vi "robot - Draw Span.vi"(4 "Color":u32(colorbox)=10079334, 6 "Center 2":cluster{"X":dbl, "Y":dbl}={"X"=50.0, "Y"=20.0}, 7 "Enhance Style":bool=TRUE, 8 "Center 1":cluster{"X":dbl, "Y":dbl}={"X"=20.0, "Y"=20.0}, 9 "Light Direction":dbl(knob)=314.8880943229338 scale=0.0..360.0 scale format="%.1f", 10 "Circle Spec":cluster{"Angle":dbl, "Height":dbl, "Ratio":dbl}={"Angle"=0.0, "Height"=10.0, "Ratio"=1.0}, 11 "Picture In":picture) -> (3 "Picture Out":picture)   [LabVIEW 2023]
doc: "Draw a single arm segment for the robot arm."
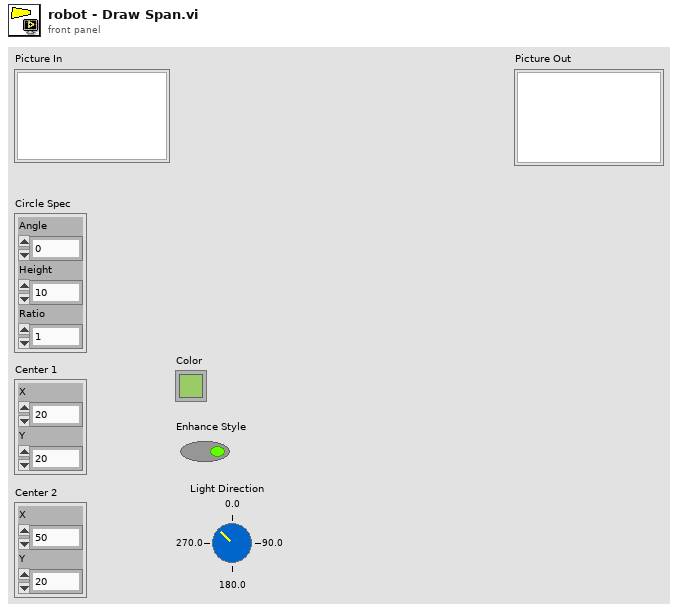
[diagram p1: front panel]
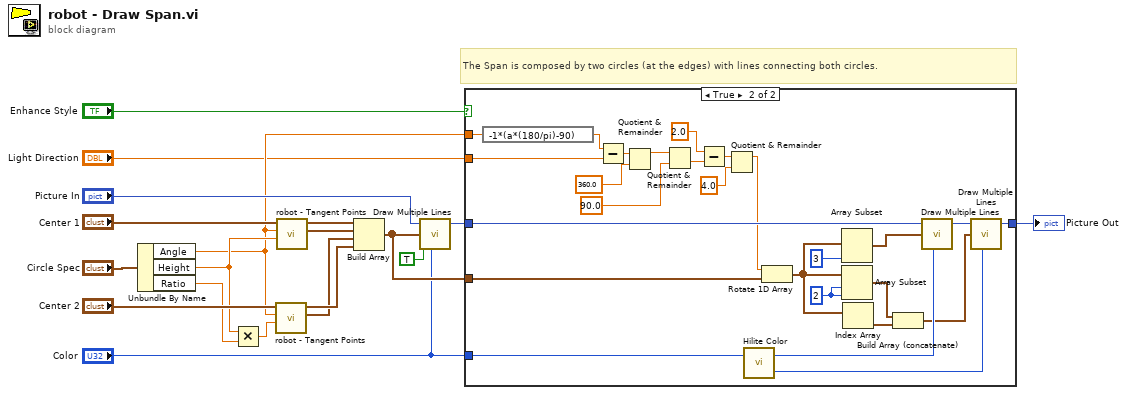
[diagram p0: block diagram]
diagram:
  # "The Span is composed by two circles (at the edges) with lines connecting both circles."
  n1 = Unbundle By Name("Circle Spec") -> ("Angle"=w3:dbl, "Height"=w4:dbl, "Ratio"=w5:dbl)
  n2 = Multiply(x=w4, y=w5) -> (x*y=w13:dbl)
  n3 = call "robot - Tangent Points.vi"("Diameter"=w13, "Rotation"=w3, "Center Point"="Center 2") -> ("Second Point"=w15:cluster{"X":dbl, "Y":dbl}, "First Point"=w18:cluster{"X":dbl, "Y":dbl})  [unwired: 7 in]
  n4 = call "robot - Tangent Points.vi"("Diameter"=w4, "Rotation"=w3, "Center Point"="Center 1") -> ("Second Point"=w19:cluster{"X":dbl, "Y":dbl}, "First Point"=w7:cluster{"X":dbl, "Y":dbl})  [unwired: 7 in]
  n5 = Build Array(w7, w19, w15, w18) -> (w9:cluster{"X":dbl, "Y":dbl}[])
  n6 = call <vilib>:"Draw Multiple Lines.vi"("picture"="Picture In", "line endpoints"=w9, "fill?(F)"=TRUE, "color(black)"="Color") -> ("new picture"=w11:picture)  [unwired: 5 in]
  n7 = case shown="True" "Enhance Style" {
    tunnel: w11 -> [w20 w46]
    tunnel: [w20 w41] -> w1
    tunnel: w9 -> [_ w36]
    tunnel: "Color" -> [_ w30]
    tunnel: w3 -> [_ w29]
    tunnel: "Light Direction" -> [_ w27]
    frame False {
    }
    frame True {
      w22 = 2
      n8 = expression code="-1*(a*(180/pi)-90)"(w29) -> (w28:dbl)
      n9 = Subtract(x=w28, y=w27) -> (x-y=w35:dbl)
      n10 = Quotient & Remainder(x=w35, y=360.0) -> (x-y*floor(x/y)=w34:dbl)  [unwired: 1 out]
      n11 = Quotient & Remainder(x=w34, y=90.0) -> (floor(x/y)=w31:dbl)  [unwired: 1 out]
      n12 = Subtract(x=2.0, y=w31) -> (x-y=w33:dbl)
      n13 = Quotient & Remainder(x=w33, y=4.0) -> (x-y*floor(x/y)=w32:dbl)  [unwired: 1 out]
      n14 = call <vilib>:"Hilite Color.vi"("Color In"=w30) -> ("Shadow"=w44:u32, "Hilite"=w45:u32)  [unwired: 1 in]
      n15 = Rotate 1D Array(1:w36, 2:w32) -> (0:w37:cluster{"X":dbl, "Y":dbl}[])
      n16 = Array Subset(array=w37, length=3) -> (w43:cluster{"X":dbl, "Y":dbl}[])  [unwired: 1 in]
      n17 = Array Subset(array=w37, index=w22, length=w22) -> (w40:cluster{"X":dbl, "Y":dbl}[])
      n18 = Index Array(array=w37) -> (element=w38:cluster{"X":dbl, "Y":dbl})  [unwired: 1 in]
      n19 = Build Array (concatenate)(w40, w38) -> (w39:cluster{"X":dbl, "Y":dbl}[])
      n20 = call <vilib>:"Draw Multiple Lines.vi"("picture"=w46, "line endpoints"=w43, "color(black)"=w45) -> ("new picture"=w42:picture)  [unwired: 6 in]
      n21 = call <vilib>:"Draw Multiple Lines.vi"("picture"=w42, "line endpoints"=w39, "color(black)"=w44) -> ("new picture"=w41:picture)  [unwired: 6 in]
    }
  }
  "Picture Out" <- w1
